vi "2016 Rush Shooter Control.vi"(8 "ballInBanner":bool, 9 "Spin up wheels button":bool, 10 "Banner ball\nin hopper":bool, 11 "Shoot button":bool) -> (0 "Shooter Wheel Speed Mode?":bool, 1 "Shooter wheel speeds":dbl, 2 "Harvester actuator back":bool, 3 "Harvester actuator front":bool)   [LabVIEW 2015]
uses:
  ArmStates.ctl
  Robot Global Data.vi
panel:
  in  "Wheel Speed":dbl=0.9 format="%#_13g"
  # "Inputs"
  # "Outputs"
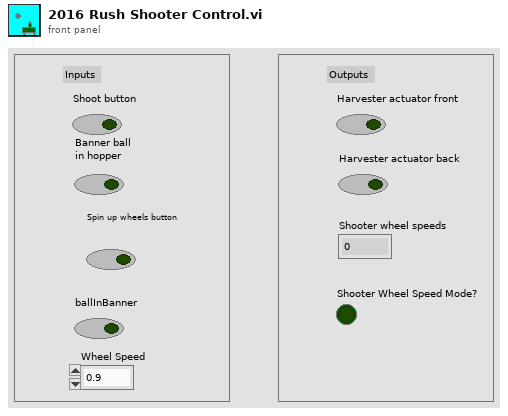
[diagram p1: front panel]
types:
  T1 = typedef "ArmStates.ctl" = enum16{"Arm Drive Position", "Shoot Position", "Roll Out", "Hic Up Rollers Off", "Draw Bridge Arm Down", "Harvest Back Down", "Harvest Hic up", "Portcullis", "Sally Door", "Harvest", "Arm Up", "Arm Down"}
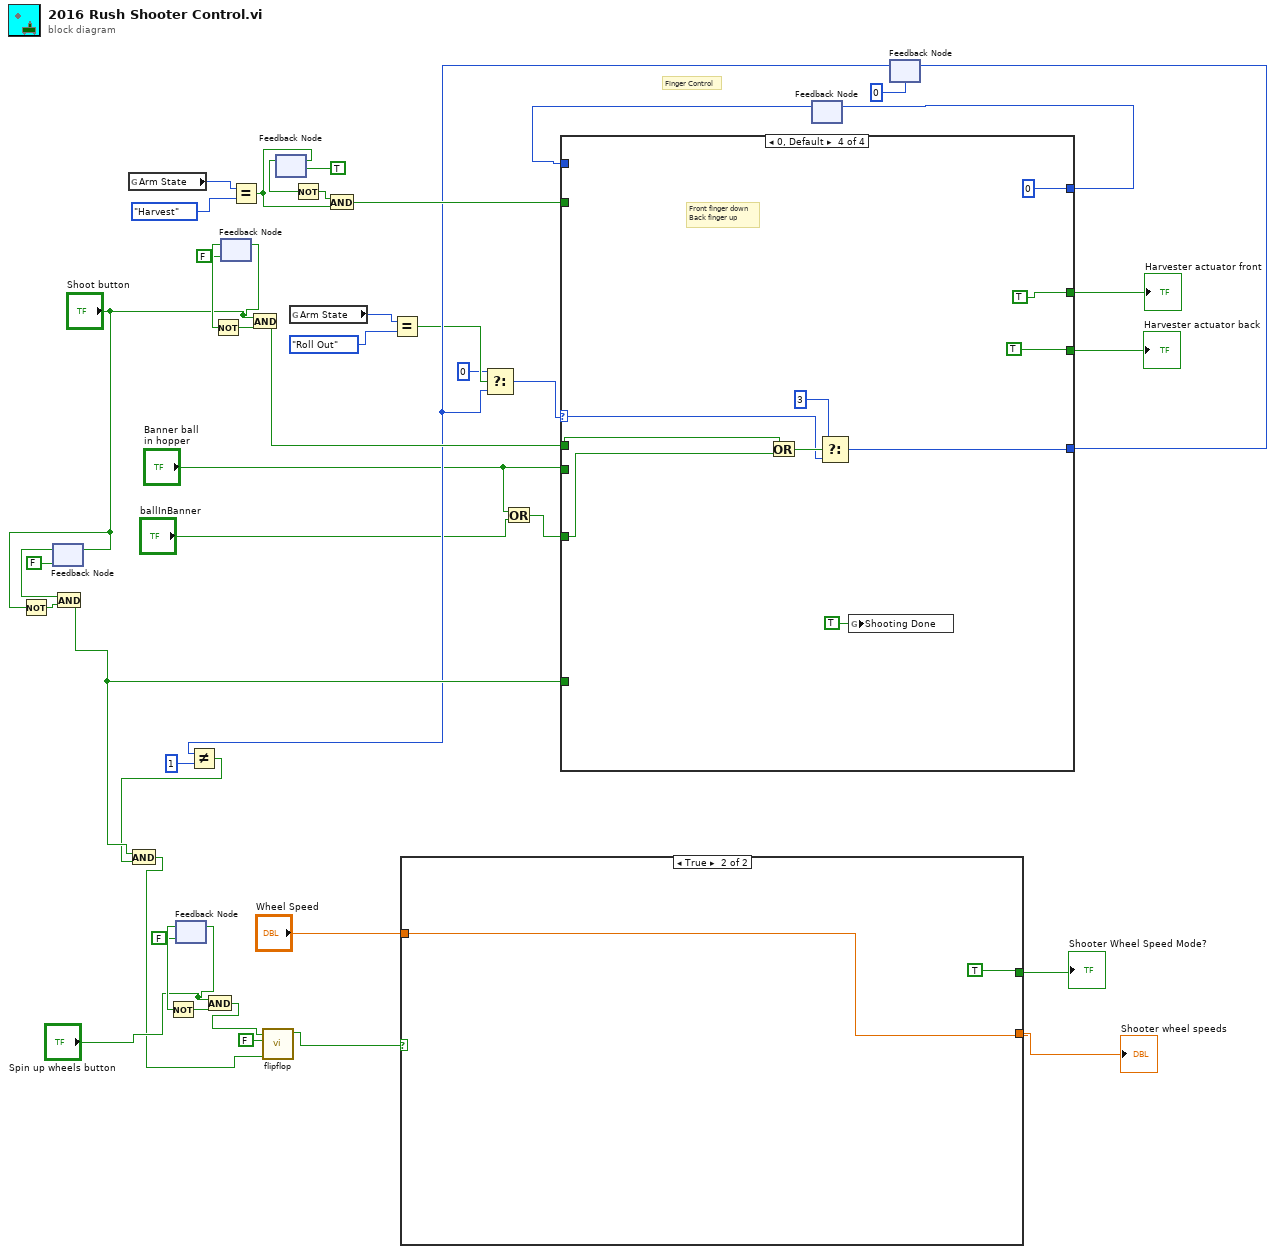
[diagram p0: block diagram]
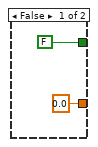
[diagram p2: hidden frame]
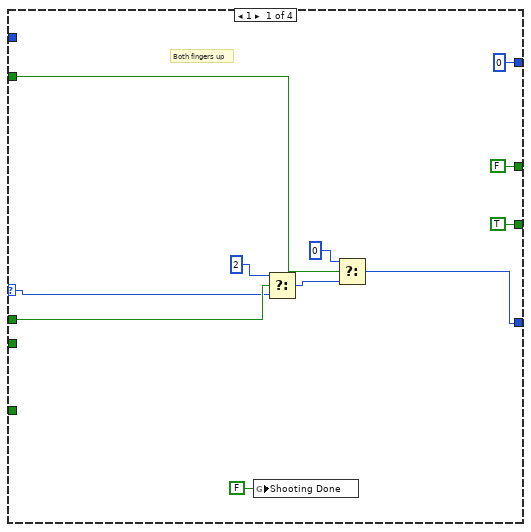
[diagram p3: hidden frame]
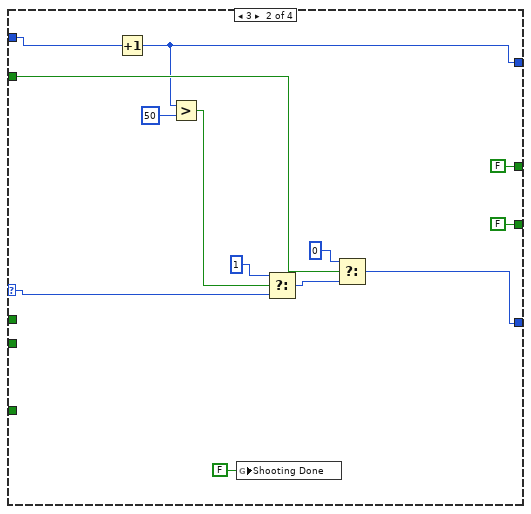
[diagram p4: hidden frame]
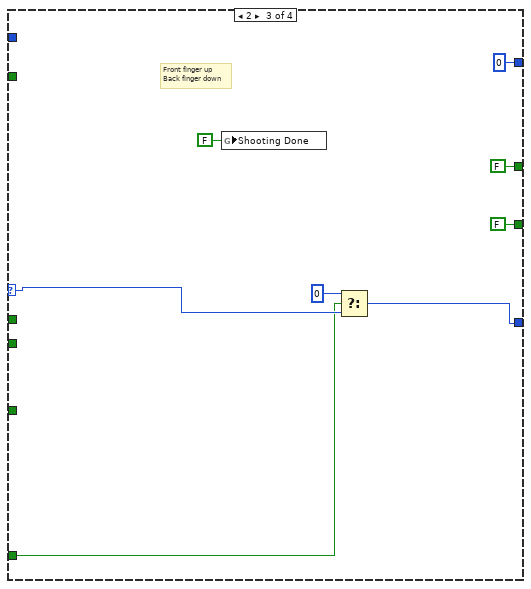
[diagram p5: hidden frame]
diagram:
  # "Finger Control"
  n1 = Not(x="Shoot button") -> (.not. x?=w36:bool)
  n2 = feedback-in #1("Shoot button") -> ()
  n3 = feedback #1(FALSE ("Shoot button")) -> (w35:bool)
  n4 = And(x=w35, y=w36) -> (x .and. y?=w23:bool)
  n5 = global read "Robot Global Data.vi" "Arm State"() -> (w18:T1)
  n6 = feedback #2(FALSE ("Shoot button")) -> (w27:bool)
  n7 = Not(x=w27) -> (.not. x?=w28:bool)
  n8 = feedback-in #2("Spin up wheels button") -> ()
  n9 = And(x="Spin up wheels button", y=w28) -> (x .and. y?=w25:bool)
  n10 = feedback-in #3("Shoot button") -> ()
  n11 = feedback #3(FALSE ("Shoot button")) -> (w31:bool)
  n12 = Not(x=w31) -> (.not. x?=w32:bool)
  n13 = Equal?(x=w18, y=ArmStates."Harvest" ("Arm State 2")) -> (x = y?=w14:bool)
  n14 = And(x="Shoot button", y=w32) -> (x .and. y?=w33:bool)
  n15 = feedback-in #4(w14) -> ()
  n16 = feedback #4(TRUE) -> (w15:bool)
  n17 = global read "Robot Global Data.vi" "Arm State"() -> (w11:T1)
  n18 = Not(x=w15) -> (.not. x?=w16:bool)
  n19 = And(x=w16, y=w14) -> (x .and. y?=w13:bool)
  n20 = Equal?(x=w11, y=ArmStates."Roll Out" ("Arm State 2")) -> (x = y?=w7:bool)
  n21 = Or(x="Banner ball\nin hopper", y="ballInBanner") -> (x .or. y?=w1:bool)
  n22 = feedback #5() -> (w4:i32)  [unwired: 1 in]
  n23 = feedback #6(0 ("t")) -> (w9:i32)
  n24 = Not Equal?(x=w9, y=1) -> (x != y?=w20:bool)
  n25 = And(x=w23, y=w20) -> (x .and. y?=w22:bool)
  n26 = call "flipflop.vi"("Overide false"=w22, "Start value"=FALSE, "flip"=w25) -> ("flop"=w42:bool)  [unwired: 8 in]
  n27 = case shown="True" w42 {
    tunnel: [0.0 ("Wheel Speed") w48] -> w38
    tunnel: "Wheel Speed" -> [_ w48]
    tunnel: [FALSE TRUE] -> w19
    frame False {
    }
    frame True {
    }
  }
  "Shooter wheel speeds" <- w38
  "Shooter Wheel Speed Mode?" <- w19
  n28 = Select(t=0, s=w7, f=w9) -> (s? t:f=w8:i32)
  n29 = case shown="0, Default" w8 {
    selector: w8 -> [w56 w70 w78 w84]
    tunnel: [FALSE FALSE FALSE TRUE] -> w44
    tunnel: [TRUE FALSE FALSE TRUE] -> w43
    tunnel: "Banner ball\nin hopper" -> [_ _ _ _]
    tunnel: w33 -> [w57 _ _ w88]
    tunnel: [w53 w67 w76 w85] -> w40
    tunnel: w23 -> [_ _ w75 _]
    tunnel: w13 -> [w52 w66 _ _]
    tunnel: w1 -> [_ _ _ w83]
    tunnel: w4 -> [_ w64 _ _]
    tunnel: [0 w63 0 0] -> w5
    frame 1 {
      # "Both fingers up"
      n30 = global write "Robot Global Data.vi" "Shooting Done"(FALSE ("Shooting Done")) -> ()
      n31 = Select(t=2, s=w57, f=w56) -> (s? t:f=w54:i32)
      n32 = Select(t=0, s=w52, f=w54) -> (s? t:f=w53:i32)
    }
    frame 3 {
      n33 = Increment(x=w64) -> (x+1=w63:i32)
      n34 = Greater?(x=w63, y=50) -> (0:w61:bool)
      n35 = global write "Robot Global Data.vi" "Shooting Done"(FALSE ("Shooting Done")) -> ()
      n36 = Select(t=1, s=w61, f=w70) -> (s? t:f=w68:i32)
      n37 = Select(t=0, s=w66, f=w68) -> (s? t:f=w67:i32)
    }
    frame 2 {
      # "Front finger up \nBack finger down"
      n38 = global write "Robot Global Data.vi" "Shooting Done"(FALSE ("Shooting Done")) -> ()
      n39 = Select(t=0, s=w75, f=w78) -> (s? t:f=w76:i32)
    }
    frame 0, Default {
      # "Front finger down\nBack finger up"
      n40 = Or(x=w88, y=w83) -> (x .or. y?=w87:bool)
      n41 = Select(t=3, s=w87, f=w84) -> (s? t:f=w85:i32)
      n42 = global write "Robot Global Data.vi" "Shooting Done"(TRUE ("Shooting Done")) -> ()
    }
  }
  "Harvester actuator front" <- w44
  "Harvester actuator back" <- w43
  n43 = feedback-in #5(w5) -> ()
  n44 = feedback-in #6(w40) -> ()
